vi "Alpha Beta Gamma Filter.vi"(6 "dt":dbl, 8 "gamma":dbl, 9 "beta":dbl, 10 "alpha":dbl, 11 "input":dbl) -> (3 "xk":dbl)   [LabVIEW 2020]
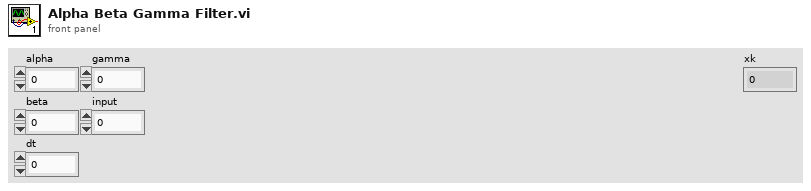
[diagram p1: front panel]
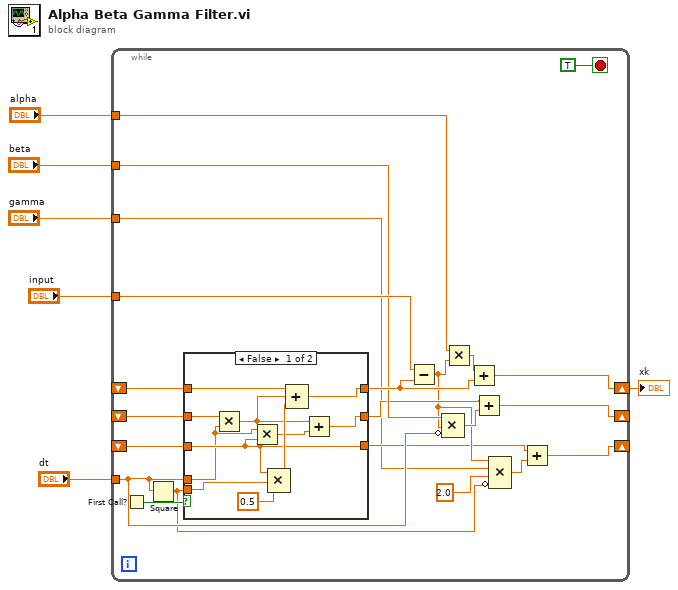
[diagram p0: block diagram]
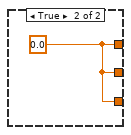
[diagram p2: hidden frame]
diagram:
  n1 = while {
    shift-right: [w19] -> w1
    shift-left: _ -> [w26]
    shift-right: [w14] -> _
    shift-left: _ -> [w25]
    shift-right: [w8] -> _
    shift-left: _ -> [w24]
    tunnel: "dt" -> [w17]
    tunnel: "input" -> [w23]
    tunnel: "alpha" -> [w21]
    tunnel: "beta" -> [w18]
    tunnel: "gamma" -> [w7]
    stop <- TRUE stop-if-true
    n2 = First Call?() -> (First Call?: T/F=w27:bool)
    n3 = Square(x=w17) -> (x^2=w13:dbl)
    n4 = case shown="False" w27 {
      tunnel: w26 -> [w39 _]
      tunnel: w25 -> [w38 _]
      tunnel: w24 -> [w33 _]
      tunnel: [w37 w40] -> w22
      tunnel: [w30 w40] -> w15
      tunnel: [w33 w40] -> w9
      tunnel: w17 -> [w32 _]
      tunnel: w13 -> [w29 _]
      frame False {
        n5 = Multiply(x=w38, y=w32) -> (x*y=w34:dbl)
        n6 = Multiply(x=w32, y=w33) -> (x*y=w31:dbl)
        n7 = Compound Arithmetic op=MULTIPLY(w33, w29, 0.5 ("value")) -> (w35:dbl)
        n8 = Compound Arithmetic op=ADD(w39, w34, w35) -> (w37:dbl)
        n9 = Add(x=w34, y=w31) -> (x+y=w30:dbl)
      }
      frame True {
        w40 = 0.0 ("input")
      }
    }
    n10 = Subtract(x=w23, y=w22) -> (x-y=w11:dbl)
    n11 = Compound Arithmetic op=MULTIPLY(w18, w11, invert w17) -> (w16:dbl)
    n12 = Multiply(x=w21, y=w11) -> (x*y=w20:dbl)
    n13 = Add(x=w20, y=w22) -> (x+y=w19:dbl)
    n14 = Add(x=w15, y=w16) -> (x+y=w14:dbl)
    n15 = Compound Arithmetic op=MULTIPLY(w11, w7, 2.0 ("value"), invert w13) -> (w10:dbl)
    n16 = Add(x=w9, y=w10) -> (x+y=w8:dbl)
  }
  "xk" <- w1
